vi "Main.vi"() -> ()   [LabVIEW 2020, in "SOL-Scorer.lvlib"]
uses:
  SOL-Scorer.lvlib
  Do Scoring Async.vi
  <vilib>/Utility/config.llb/Read Key (Double).vi
  <vilib>/Utility/config.llb/NI_LVConfig.lvlib
panel:
  out "Run Time":dbl format="%<%M:%S>t"
  in  "Abort":bool
  out "LLB":path
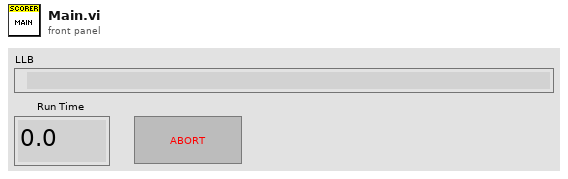
[diagram p1: front panel]
types:
  T1 = enum32{"Bad", "Idle", "Run top level", "Running"}
  T2 = typedef "NI_LVConfig.lvlib/Config Data RefNum.ctl" = refnum<k1>
  T3 = typedef "SoL Scoring.lvlib/Score.ctl" = cluster{"Overall":dbl, "Categories":T4[]}
  T4 = typedef "SoL Scoring.lvlib/Score Entry.ctl" = cluster{"Category":string, "Value":dbl}
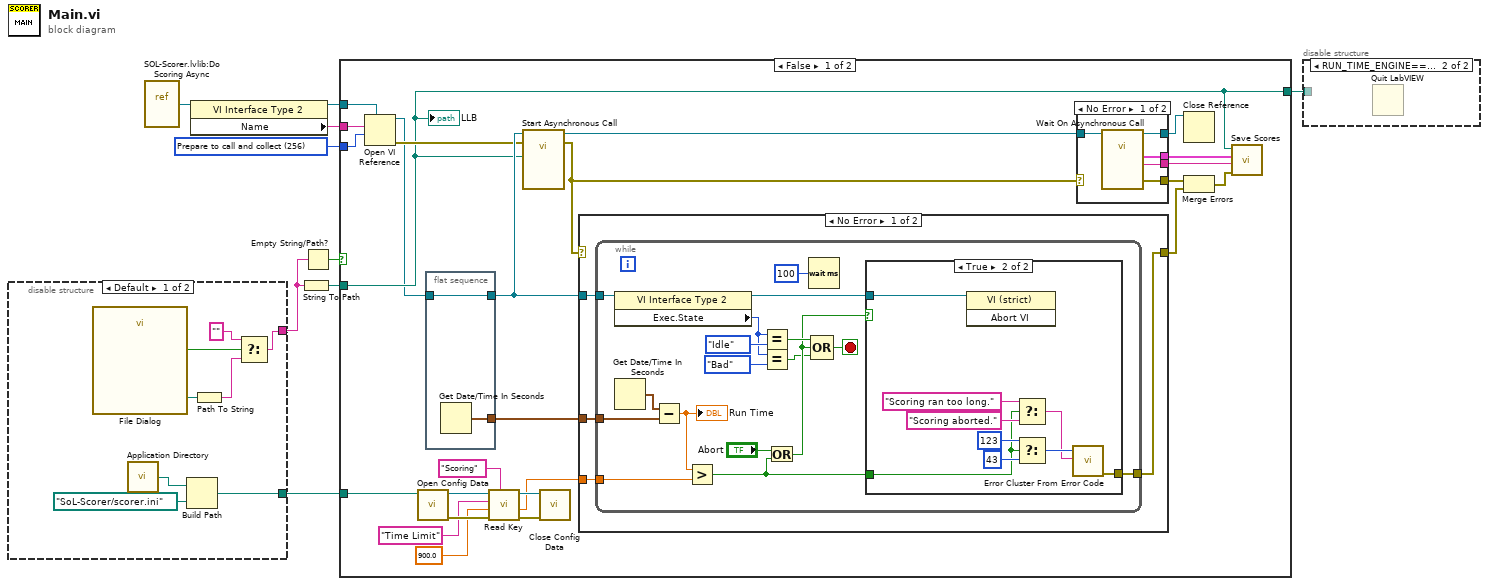
[diagram p0: block diagram]
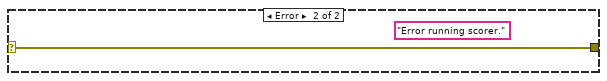
[diagram p4: hidden frame]
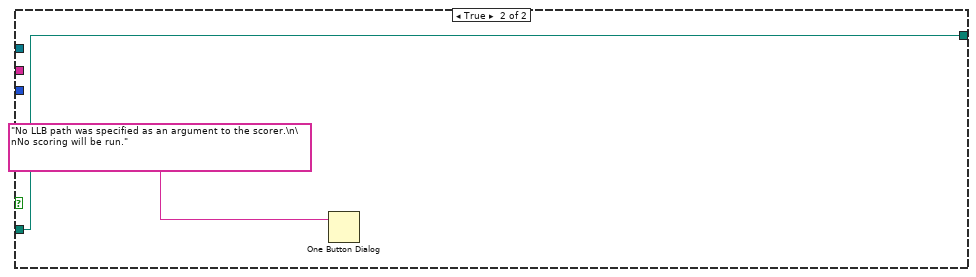
[diagram p5: hidden frame]
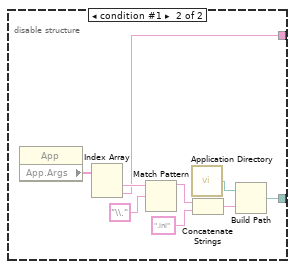
[diagram p6: hidden frame]
diagram:
  w8 = 256 items=["Record modifications"=1, "Open templates for editing"=2, "Prompt user to save"=4, "Prepare for reentrant run"=8, "Prompt to find missing subVIs"=16, "Hide loading dialog box"=32, "Enable simultaneous calls"=64, "Prepare to call and forget"=128, "Simultaneous call and forget"=192, "Prepare to call and collect"=256, "Simultaneous call and collect"=320]
  n1 = disable-structure shown="Default" {
    disable-tunnel: [w11 w24] -> w2
    disable-tunnel: [w16 w18] -> w1
    frame condition #0 (active) {
      n2 = call "File Dialog"() -> ("selected path"=w14:path, "cancelled"=w13:bool)  [unwired: 12 in, 2 out]
      n3 = call <vilib>:"Application Directory.vi"() -> ("Application Directory"=w17:path)
      n4 = Build Path(base path=w17, name or relative path=path "SoL-Scorer/scorer.ini") -> (appended path=w16:path)
      n5 = Path To String(path=w14) -> (string=w12:string)
      n6 = Select(t="", s=w13, f=w12) -> (s? t:f=w11:string)
    }
    frame condition #1 {
      n7 = property class="App"() -> ("App.Args"=w26:string[])  [unwired: 2 in, 2 out]
      n8 = Index Array(array=w26) -> (element #1=w25:string, element #2=w24:string)  [unwired: 2 in]
      n9 = Match Pattern(string=w25, regular expression="\\.") -> (before substring=w19:string)  [unwired: 1 in, 3 out]
      n10 = call <vilib>:"Application Directory.vi"() -> ("Application Directory"=w22:path)
      n11 = Concatenate Strings(w19, ".ini" ("string")) -> (w21:string)
      n12 = Build Path(base path=w22, name or relative path=w21) -> (appended path=w18:path)
    }
  }
  n13 = vi-ref "SOL-Scorer.lvlib:Do Scoring Async.vi"() -> (w6:refnum<vi>)
  n14 = property class="VI Interface Type 2"(reference=w6) -> (reference out=w9:refnum<vi>, "Name"=w7:string)  [unwired: 1 in, 1 out]
  n15 = String To Path(string=w2) -> (path=w5:path)
  n16 = Empty String/Path?(string/path=w2) -> (empty?=w4:bool)
  n17 = case shown="False" w4 {
    tunnel: w9 -> [w51 _]
    tunnel: w8 -> [w50 _]
    tunnel: w7 -> [w49 _]
    tunnel: w5 -> [w33 w92]
    tunnel: [w33 w92] -> w3
    tunnel: w1 -> [w32 _]
    frame False {
      n18 = Open VI Reference(type specifier VI Refnum (for type only)=w51, vi path=w49, options=w50) -> (vi reference=w31:refnum<vi>, error out=w37:errorcluster)  [unwired: 3 in]
      n19 = call <vilib>:"Open Config Data.vi"("configuration file path"=w32) -> ("error out"=w45:errorcluster, "refnum"=w46:T2)  [unwired: 8 in, 1 out]
      n20 = flat-sequence {
        tunnel: w31 -> [w53]
        tunnel: [w53] -> w48
        tunnel: [w52] -> w47
        frame #0 {
          n21 = Get Date/Time In Seconds() -> (seconds since 1Jan1904=w52:timestamp)
        }
      }
      n22 = call-poly <vilib>:"Read Key.vi"("section"="Scoring", "error in (no error)"=w45, "default value"=900.0 ("y"), "key"="Time Limit" ("section"), "refnum"=w46) -> ("error out"=w40:errorcluster, "value"=w39:dbl, "refnum out"=w41:T2)  [unwired: 3 in, 1 out]
      n23 = call-by-ref "Start Asynchronous Call"(reference=w48, error in=w37, "Submission LLB"=w33) -> (reference out=w38:refnum<vi>, error out=w29:errorcluster)  [unwired: 8 in, 3 out]
      n24 = call <vilib>:"Close Config Data.vi"("error in (no error)"=w40, "refnum"=w41) -> ()  [unwired: 8 in, 2 out]
      n25 = case shown="No Error" w29 {
        selector: w29 -> [_ w91]
        tunnel: w48 -> [w64 _]
        tunnel: w47 -> [w63 _]
        tunnel: w39 -> [w62 _]
        tunnel: [w61 w91] -> w27
        frame No Error {
          n26 = while {
            tunnel: w64 -> [w76]
            tunnel: w63 -> [w80]
            tunnel: w62 -> [w77]
            tunnel: [w71] -> w61
            stop <- w73 stop-if-true
            n27 = property class="VI Interface Type 2"(reference=w76) -> (reference out=w72:refnum<vi>, "Exec.State"=w66:T1)  [unwired: 1 in, 1 out]
            n28 = Get Date/Time In Seconds() -> (seconds since 1Jan1904=w79:timestamp)
            n29 = Subtract(x=w79, y=w80) -> (x-y=w78:dbl)
            "Run Time" <- w78
            n30 = Greater?(x=w78, y=w77) -> (0:w68:bool)
            n31 = Equal?(x=w66, y=T1."Idle") -> (x = y?=w74:bool)
            n32 = Equal?(x=w66, y=T1."Bad") -> (x = y?=w65:bool)
            n33 = Or(x="Abort", y=w68) -> (x .or. y?=w69:bool)
            n34 = Wait (ms)(milliseconds to wait=u32 100) -> ()  [unwired: 1 out]
            n35 = Compound Arithmetic op=OR(w74, w69, w65) -> (w73:bool)
            n36 = case shown="True" w69 {
              tunnel: w72 -> [_ w90]
              tunnel: [_ w89] -> w71
              tunnel: w68 -> [_ w83]
              frame False {
              }
              frame True {
                n37 = invoke class="VI (strict)" method="Abort VI"(reference=w90) -> ()  [unwired: 2 in, 3 out]
                n38 = Select(t="Scoring ran too long." ("error message (\"\")"), s=w83, f="Scoring aborted." ("error message (\"\")")) -> (s? t:f=w82:string)
                n39 = Select(t=123 ("error code (0)"), s=w83, f=43 ("error code (0)")) -> (s? t:f=w86:i32)
                n40 = call <vilib>:"Error Cluster From Error Code.vi"("error message (\"\")"=w82, "error code (0)"=w86) -> ("error out"=w89:errorcluster)  [unwired: 7 in]
              }
            }
          }
        }
        frame Error {
          (unwired) "Error running scorer." ("error message (\"\")")
        }
      }
      n41 = case shown="No Error" w29 {
        selector: w29 -> [_ w60]
        tunnel: w38 -> [w58 w59]
        tunnel: [w57 _] -> w36
        tunnel: [w56 _] -> w35
        tunnel: [w55 w60] -> w34
        tunnel: [w54 w59] -> w30
        frame No Error {
          n42 = call-by-ref "Wait On Asynchronous Call"(reference=w58) -> (reference out=w54:refnum<vi>, "error out"=w55:errorcluster, "Test Summary"=w56:string, "Score"=w57:T3)  [unwired: 10 in, 1 out]
        }
        frame Error {
        }
      }
      n43 = Close Reference(reference=w30) -> ()  [unwired: 1 in, 1 out]
      n44 = Merge Errors(w34, w27) -> (w28:errorcluster)
      n45 = call "Save Scores.vi"("error in (no error)"=w28, "Test Summary"=w35, "Score"=w36, "LLB Path"=w33) -> ()  [unwired: 8 in]
      "LLB" <- w33
    }
    frame True {
      n46 = One Button Dialog(message="No LLB path was specified as an argument to the scorer.\n\nNo scoring will be run.") -> ()  [unwired: 1 in, 1 out]
    }
  }
  n47 = disable-structure shown="RUN_TIME_ENGINE==True" {
    disable-tunnel: w3 -> [_ _]
    frame condition #0 (active) {
    }
    frame condition #1 {
      n48 = Quit LabVIEW() -> ()  [unwired: 1 in]
    }
  }
